vi "Bundle_Split First and Other Strings.vi"(7 "Strings In":string[](array[string])) -> (4 "First String":string, 6 "One or More Other Strings":bool, 8 "Other Strings":string[](array[string]))   [LabVIEW 2025]
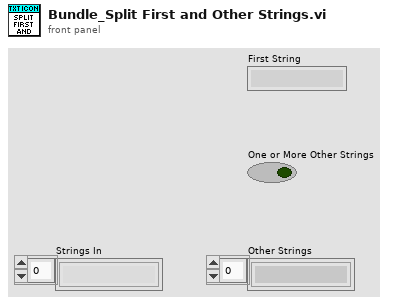
[diagram p1: front panel]
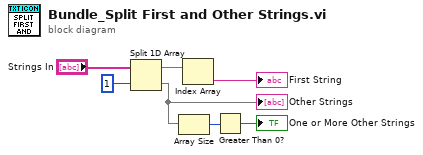
[diagram p0: block diagram]
diagram:
  n1 = Split 1D Array(array="Strings In", index=1) -> (first subarray=w3:string[], second subarray=w5:string[])
  "Other Strings" <- w5
  n2 = Array Size(array=w5) -> (size(s)=w6:i32)
  n3 = Index Array(array=w3) -> (element=→"First String":string)  [unwired: 1 in]
  n4 = Greater Than 0?(x=w6) -> (x > 0?=→"One or More Other Strings":bool)
